vi "User32_FindWindowA.vi"(8 "error in (no error)":errorcluster, 11 "lpszWindowName":string) -> (0 "error out":errorcluster, 3 "hWnd":u64)   [LabVIEW 2017]
uses:
  user32.dll
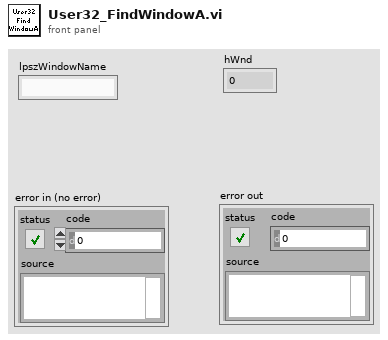
[diagram p1: front panel]
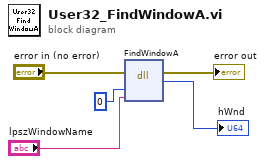
[diagram p0: block diagram]
diagram:
  n1 = dll-call lib="user32.dll" fn="FindWindowA"(error in="error in (no error)", "lpszClassName"=u32 0, "lpszWindowName"="lpszWindowName") -> (error out=→"error out":errorcluster, "hWnd"=→"hWnd":u64)  [unwired: 4 in, 1 out]
